vi "Periodic Tasks.vi"(8 "error in":errorcluster) -> ()   [LabVIEW 2012]
doc: "This VI runs in parallel to other tasks. It can contain as many user-defined periodic loops as you need. These can carry out PID or other sorts of timed response."
uses:
  <vilib>/Rock Robotics/WPI/Compressor/WPI_CompressorGetSetRefNum.vi
  <vilib>/Rock Robotics/WPI/RobotDrive/WPI_RobotDriveGetSetRefNum.vi
  <vilib>/Rock Robotics/WPI/Joystick/WPI_JoystickGetSetRefNum.vi
  <vilib>/Rock Robotics/WPI/Solenoid/Deprecated/WPI_SolenoidSetBool.vi
panel:
  in  "Slow Turn":dbl
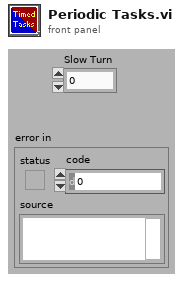
[diagram p1: front panel]
types:
  T1 = typedef "WPI_RobotDriveDevRef.ctl" = cluster{"DevStatus":errorcluster, "Motors[]":T2[], "Square Inputs":bool, "Max Output":dbl, "Isochronous":bool}
  T2 = typedef "WPI_MotorControlDeviceRef.ctl" = cluster{"DeviceStatus":errorcluster, "Type":enum16{"PWM", "CAN"}, "PWM":cluster{"Digital Module":T3, "PWM Channel":T4, "DeadBand":T5}, "CAN":cluster{"Device Number":u8, "Control Mode":T6, "Semaphore":T7, "Max Vout":dbl}, "Invert":bool, "TransformRef":T8, "InvTransformRef":T8}
  T3 = typedef "FPGA_TypedefDigitalModule.ctl" = enum16{"Digital Module 1", "Digital Module 2"}
  T4 = typedef "FPGA_DIOPWMChannel.ctl" = enum8{"PWM 1", "PWM 2", "PWM 3", "PWM 4", "PWM 5", "PWM 6", "PWM 7", "PWM 8", "PWM 9", "PWM 10", "Invalid"}
  T5 = typedef "WPI_PWMDeadband.ctl" = cluster{"Name":string, "maxPositivePwm":i32, "minPositivePwm":i32, "centerPwm":i32, "maxNegativePwm":i32, "minNegativePwm":i32, "angularRange":u16}
  T6 = typedef "WPI_CANJaguar_ControlMode.ctl" = enum8{"Percent VBus", "Current", "Speed", "Position", "Voltage"}
  T7 = typedef "Semaphore RefNum" = refnum<k1>
  T8 = typedef "WPI_PWMTransform_ConPane.ctl" = refnum<vi>
  T9 = typedef "WPI_JoystickDevRef.ctl" = cluster{"Device":T10}
  T10 = typedef "WPI_JoystickDeviceEnum.ctl" = enum16{"USB 1", "USB 2", "USB 3", "USB 4", "Kinect 1", "Kinect 2"}
  T11 = cluster{"JoystickDevRef":T9, "RobotDriveDevRef":T1, "MotorControlDevRef":T2}
  T12 = typedef "WPI_SolenoidDevRef.ctl" = cluster{"DevStatus":errorcluster, "Solenoid Module":T13, "Forward Solenoid Channel":T14, "Reverse Solenoid Channel":T14}
  T13 = typedef "FPGA_TypedefSolenoidModule.ctl" = enum16{"Solenoid Module 1", "Solenoid Module 2"}
  T14 = typedef "WPI_SolenoidChannel.ctl" = enum8{"Solenoid 1", "Solenoid 2", "Solenoid 3", "Solenoid 4", "Solenoid 5", "Solenoid 6", "Solenoid 7", "Solenoid 8", "Invalid"}
  T15 = typedef "WPI_CompressorDevRef.ctl" = cluster{"DevStatus":errorcluster, "DigitalInputDevRef":T16, "RelayDevRef":T18}
  T16 = typedef "WPI_DigitalInputDevRef.ctl" = cluster{"DevStatus":errorcluster, "DIO Channel":T17, "Digital Module":T3}
  T17 = typedef "FPGA_DIOChannel.ctl" = enum8{"DIO 1", "DIO 2", "DIO 3", "DIO 4", "DIO 5", "DIO 6", "DIO 7", "DIO 8", "DIO 9", "DIO 10", "DIO 11", "DIO 12", "DIO 13", "DIO 14", "Invalid"}
  T18 = typedef "WPI_RelayDevRef.ctl" = cluster{"DevStatus":errorcluster, "Relay Channel":T19, "Digital Module":T3, "Relay Direction":T20}
  T19 = typedef "FPGA_DIORelayChannel.ctl" = enum8{"Relay 1", "Relay 2", "Relay 3", "Relay 4", "Relay 5", "Relay 6", "Relay 7", "Relay 8", "Invalid"}
  T20 = typedef "WPI_RelayDirection.ctl" = enum16{"Both directions", "Forward only", "Reverse only"}
  T21 = typedef "WPI_DigitalOutputDevRef.ctl" = cluster{"Digital Module":T3, "DIO Channel":T17, "DevStatus":errorcluster}
  T22 = typedef "WPI_JoystickButtonState.ctl" = cluster{"Button 1":bool, "Button 2":bool, "Button 3":bool, "Button 4":bool, "Button 5":bool, "Button 6":bool, "Button 7":bool, "Button 8":bool, "Button 9":bool, "Button 10":bool, "Button 11":bool, "Button 12":bool}
  T23 = cluster{"axis 1 (x)":dbl, "axis 2 (y)":dbl, "axis 3 (throttle)":dbl, "axis 4":dbl, "axis 5":dbl, "axis 6":dbl}
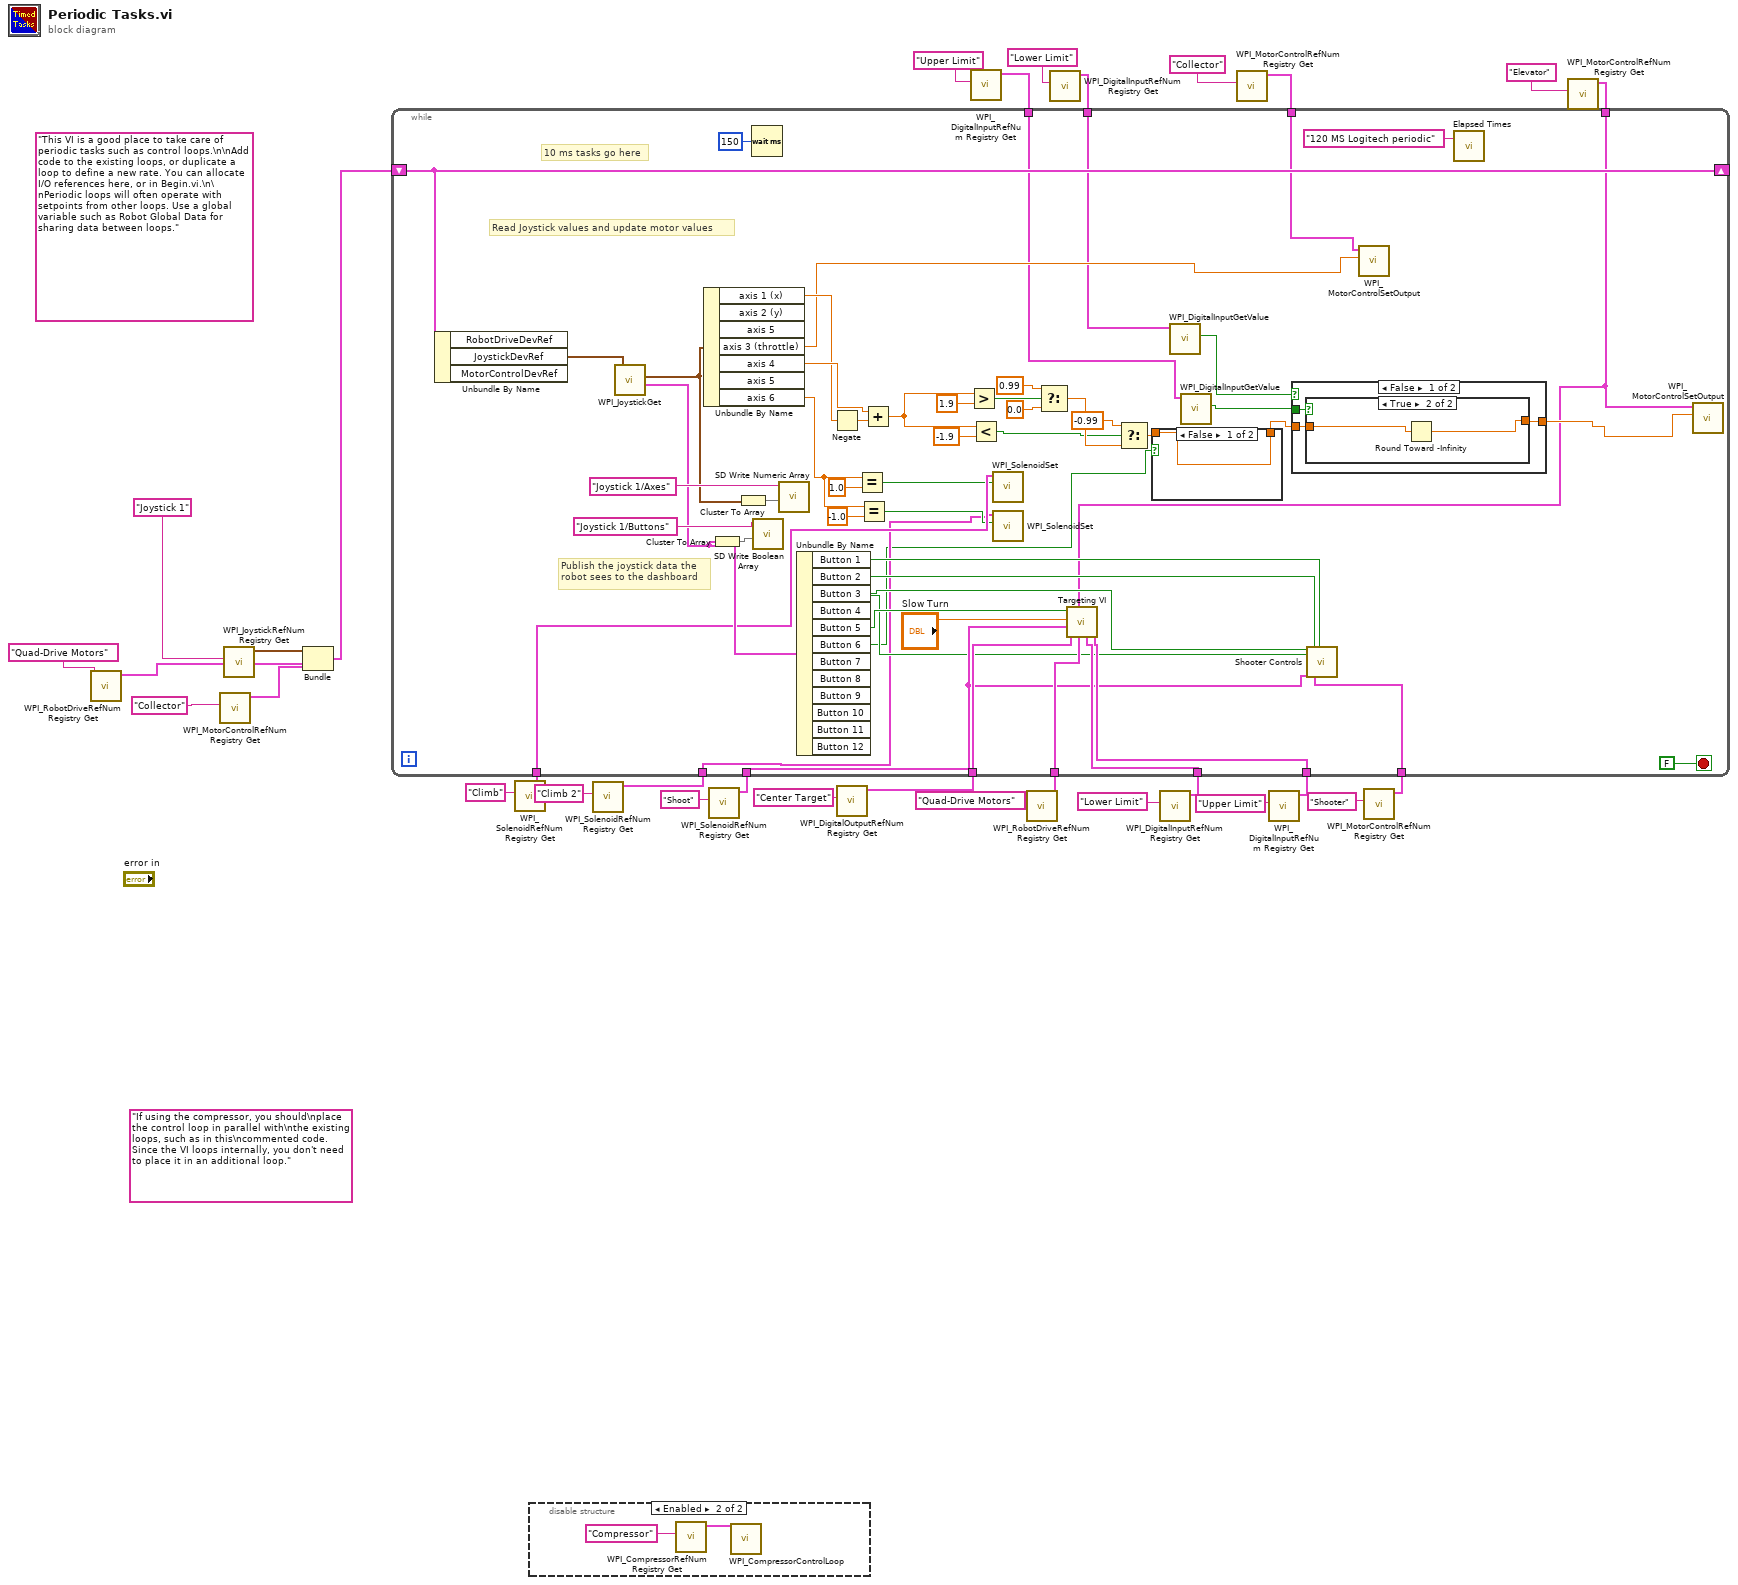
[diagram p0: block diagram]
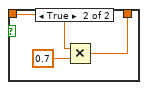
[diagram p3: hidden frame]
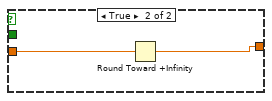
[diagram p5: hidden frame]
diagram:
  (unwired) "If using the compressor, you should\nplace the control loop in parallel with\nthe existing loops, such as in this\ncommented code. Since the VI loops internally, you don't need to place it in an additional loop."
  (unwired) "This VI is a good place to take care of periodic tasks such as control loops.\n\nAdd code to the existing loops, or duplicate a loop to define a new rate. You can allocate I/O references here, or in Begin.vi.\n\nPeriodic loops will often operate with setpoints from other loops. Use a global variable such as Robot Global Data for sharing data between loops."
  n1 = call <vilib>:"WPI_RobotDriveRefNum Registry Get.vi"("refnum name"="Quad-Drive Motors") -> ("RobotDriveDevRef"=w28:T1)  [unwired: 1 in, 9 out]
  n2 = call <vilib>:"WPI_MotorControlRefNum Registry Get.vi"("refnum name"="Collector") -> ("MotorControlDevRef"=w25:T2)  [unwired: 9 in, 1 out]
  n3 = call <vilib>:"WPI_JoystickRefNum Registry Get.vi"("refnum name"="Joystick 1") -> ("JoystickDevRef"=w29:T9)  [unwired: 1 in, 9 out]
  n4 = Bundle("JoystickDevRef"=w29, "RobotDriveDevRef"=w28, "MotorControlDevRef"=w25) -> (w27:T11)  [unwired: 1 out]
  n5 = call <vilib>:"WPI_SolenoidRefNum Registry Get.vi"("refnum name"="Climb") -> ("SolenoidDevRef"=w3:T12)  [unwired: 9 in, 1 out]
  n6 = disable-structure shown="Enabled" {
    frame Disabled {
    }
    frame Enabled {
      n7 = call <vilib>:"WPI_CompressorRefNum Registry Get.vi"("refnum name"="Compressor") -> ("CompressorDevRef"=w33:T15)  [unwired: 9 in, 1 out]
      n8 = call <vilib>:"WPI_CompressorControlLoop.vi"("CompressorDevRef"=w33) -> ()  [unwired: 11 in]
    }
  }
  n9 = call <vilib>:"WPI_SolenoidRefNum Registry Get.vi"("refnum name"="Climb 2") -> ("SolenoidDevRef"=w1:T12)  [unwired: 9 in, 1 out]
  n10 = call <vilib>:"WPI_SolenoidRefNum Registry Get.vi"("refnum name"="Shoot") -> ("SolenoidDevRef"=w11:T12)  [unwired: 9 in, 1 out]
  n11 = call <vilib>:"WPI_DigitalOutputRefNum Registry Get.vi"("refnum name"="Center Target") -> ("DigitalOutputDevRef"=w15:T21)  [unwired: 9 in, 1 out]
  n12 = call <vilib>:"WPI_DigitalInputRefNum Registry Get.vi"("refnum name"="Upper Limit") -> ("DigitalInputDevRef"=w21:T16)  [unwired: 9 in, 1 out]
  n13 = call <vilib>:"WPI_RobotDriveRefNum Registry Get.vi"("refnum name"="Quad-Drive Motors") -> ("RobotDriveDevRef"=w13:T1)  [unwired: 1 in, 9 out]
  n14 = call <vilib>:"WPI_DigitalInputRefNum Registry Get.vi"("refnum name"="Lower Limit") -> ("DigitalInputDevRef"=w23:T16)  [unwired: 9 in, 1 out]
  n15 = call <vilib>:"WPI_DigitalInputRefNum Registry Get.vi"("refnum name"="Lower Limit") -> ("DigitalInputDevRef"=w8:T16)  [unwired: 9 in, 1 out]
  n16 = call <vilib>:"WPI_MotorControlRefNum Registry Get.vi"("refnum name"="Collector") -> ("MotorControlDevRef"=w17:T2)  [unwired: 9 in, 1 out]
  n17 = call <vilib>:"WPI_DigitalInputRefNum Registry Get.vi"("refnum name"="Upper Limit") -> ("DigitalInputDevRef"=w7:T16)  [unwired: 9 in, 1 out]
  n18 = call <vilib>:"WPI_MotorControlRefNum Registry Get.vi"("refnum name"="Shooter") -> ("MotorControlDevRef"=w5:T2)  [unwired: 9 in, 1 out]
  n19 = call <vilib>:"WPI_MotorControlRefNum Registry Get.vi"("refnum name"="Elevator") -> ("MotorControlDevRef"=w19:T2)  [unwired: 9 in, 1 out]
  n20 = while {
    shift-right: [w81] -> _
    shift-left: w27 -> [w81]
    tunnel: w23 -> [w54]
    tunnel: w21 -> [w53]
    tunnel: w19 -> [w50]
    tunnel: w17 -> [w52]
    tunnel: w15 -> [w51]
    tunnel: w13 -> [w49]
    tunnel: w11 -> [w45]
    tunnel: w8 -> [w48]
    tunnel: w7 -> [w47]
    tunnel: w5 -> [w46]
    tunnel: w3 -> [w43]
    tunnel: w1 -> [w37]
    stop <- FALSE stop-if-true
    # "Publish the joystick data the\nrobot sees to the dashboard"
    # "Read Joystick values and update motor values"
    # "10 ms tasks go here"
    n21 = Unbundle By Name(w81) -> ("JoystickDevRef"=w80:T9)  [unwired: 2 out]
    n22 = call <vilib>:"WPI_JoystickGet.vi"("JoystickDevRef"=w80) -> ("Buttons"=w77:T22, "Axes"=w79:T23)  [unwired: 4 in, 1 out]
    n23 = Unbundle By Name(w79) -> ("axis 1 (x)"=w59:dbl, "axis 3 (throttle)"=w55:dbl, "axis 4"=w61:dbl, "axis 6"=w41:dbl)  [unwired: 3 out]
    n24 = Cluster To Array(cluster=w77) -> (array=w78:bool[])
    n25 = Cluster To Array(cluster=w79) -> (array=w83:dbl[])
    n26 = Wait (ms)(milliseconds to wait=u32 150) -> ()  [unwired: 1 out]
    n27 = call <vilib>:"SD Write Boolean Array.vi"("Boolean Array"=w78, "Name"="Joystick 1/Buttons") -> ()  [unwired: 8 in, 2 out]
    n28 = call <vilib>:"SD Write Numeric Array.vi"("Numeric Array"=w83, "Name"="Joystick 1/Axes") -> ()  [unwired: 8 in, 2 out]
    n29 = Unbundle By Name(w77) -> ("Button 1"=w72:bool, "Button 2"=w73:bool, "Button 3"=w74:bool, "Button 4"=w44:bool, "Button 5"=w75:bool, "Button 6"=w34:bool)  [unwired: 6 out]
    n30 = Negate(x=w59) -> (-x=w60:dbl)
    n31 = Equal?(x=w41, y=1.0) -> (x = y?=w39:bool)
    n32 = Equal?(x=w41, y=-1.0) -> (x = y?=w38:bool)
    n33 = Add(x=w61, y=w60) -> (x+y=w70:dbl)
    n34 = Greater?(x=w70, y=1.9) -> (0:w67:bool)
    n35 = Less?(x=w70, y=-1.9) -> (x < y?=w62:bool)
    n36 = call-poly <vilib>:"WPI_SolenoidSet.vi"("Value"=w39, "SolenoidDevRef"=w43) -> ()  [unwired: 8 in, 2 out]
    n37 = call-poly <vilib>:"WPI_SolenoidSet.vi"("Value"=w38, "SolenoidDevRef"=w37) -> ()  [unwired: 8 in, 2 out]
    n38 = Select(t=0.99, s=w67, f=0.0) -> (s? t:f=w66:dbl)
    n39 = call "Targeting VI.vi"("Upper Limit"=w47, "Lower Limit"=w48, "RobotDriveDevRef"=w49, "Elevator Control"=w50, "DO 14 LED"=w51, "Shoot"=w45, "slow turn"="Slow Turn", "Aim Button"=w75) -> ()  [unwired: 4 in]
    n40 = Select(t=-0.99, s=w62, f=w66) -> (s? t:f=w35:dbl)
    n41 = case shown="False" w34 {
      tunnel: [w87 w89] -> w36
      tunnel: w35 -> [w87 w90]
      frame False {
      }
      frame True {
        n42 = Multiply(x=w90, y=0.7) -> (x*y=w89:dbl)
      }
    }
    n43 = call <vilib>:"WPI_DigitalInputGetValue.vi"("DigitalInputDevRef"=w54) -> ("Value"=w58:bool)  [unwired: 8 in, 2 out]
    n44 = call <vilib>:"WPI_DigitalInputGetValue.vi"("DigitalInputDevRef"=w53) -> ("Value"=w56:bool)  [unwired: 8 in, 2 out]
    n45 = case shown="False" w58 {
      tunnel: w36 -> [w93 w97]
      tunnel: [w92 w98] -> w57
      tunnel: w56 -> [w91 _]
      frame False {
        n46 = case shown="True" w91 {
          tunnel: w93 -> [w94 w95]
          tunnel: [w94 w96] -> w92
          frame False {
          }
          frame True {
            n47 = Round Toward -Infinity(1:w95) -> (0:w96:dbl)
          }
        }
      }
      frame True {
        n48 = Round Toward +Infinity(x=w97) -> (ceil(x): smallest int >= x=w98:dbl)
      }
    }
    n49 = call "Shooter Controls.vi"("X Button (shooter on, slow)"=w74, "Y button (Manual Shot)"=w44, "Shoot"=w45, "B button (Shooter Off)"=w73, "Shooter"=w46, "A Button (Shooter on, Full)"=w72) -> ()  [unwired: 14 in]
    n50 = call <vilib>:"WPI_MotorControlSetOutput.vi"("Output"=w55, "MotorControlDevRef"=w52) -> ()  [unwired: 7 in, 3 out]
    n51 = call "Elapsed Times.vi"("Call Name"="120 MS Logitech periodic") -> ()  [unwired: 2 in, 1 out]
    n52 = call <vilib>:"WPI_MotorControlSetOutput.vi"("Output"=w57, "MotorControlDevRef"=w50) -> ()  [unwired: 7 in, 3 out]
  }
